vi "OE1022_Configure Ref Phase.vi"(7 "OE1022_Configure Ref Phase":T1={"Reference Source"=0, "Sweep Mode"=0, "Start Frequency(Hz)"=1000.0, "Stop Frequency(Hz)"=90000.0, "Linear Step Frequency(Hz)"=1000.0, "Log Step Percent(%)"=10.0, "Step Time(ms)"=1000, "Sweep Run Mode"=0, "Internal Frequency(Hz)"=1000.0, "Phase  (degree)"=0.0, "External Ref Trigger"=0} {"External Ref Trigger" items=["TTL Rising Edge", "TTL Falling Edge", "Sine Zero Crossing"]; "Phase  (degree)" min=-180.0 max=180.0 format="%.2f"; "Internal Frequency(Hz)" min=0.001 max=102000.0 format="%#.3f"; "Sweep Run Mode" items=["Stop", "Singal", "Loop"]; "Step Time(ms)" min=1 max=100000; "Log Step Percent(%)" min=0.0 max=100.0 format="%#.2g"; "Linear Step Frequency(Hz)" min=0.001 max=102000.0; "Stop Frequency(Hz)" min=0.001 max=102000.0 format="%#.3f"; "Start Frequency(Hz)" min=0.001 max=102000.0 format="%#.3f"; "Sweep Mode" items=["Linear", "Log"]; "Reference Source" items=["External", "Internal", "Internal Sweep"]}, 8 "Error in (no error)":errorcluster caption="error out（no error）", 9 "Remote Mode":u16(ring) items=["USB"=0, "GPIB"=2], 11 "VISA resource name":refnum<visa-resource-name>) -> (0 "Error out":errorcluster caption="error out", 1 "Output String":string, 3 "VISA resource  out":refnum<visa-resource-name>)   [LabVIEW 2011]
panel:
  out "字符串":string
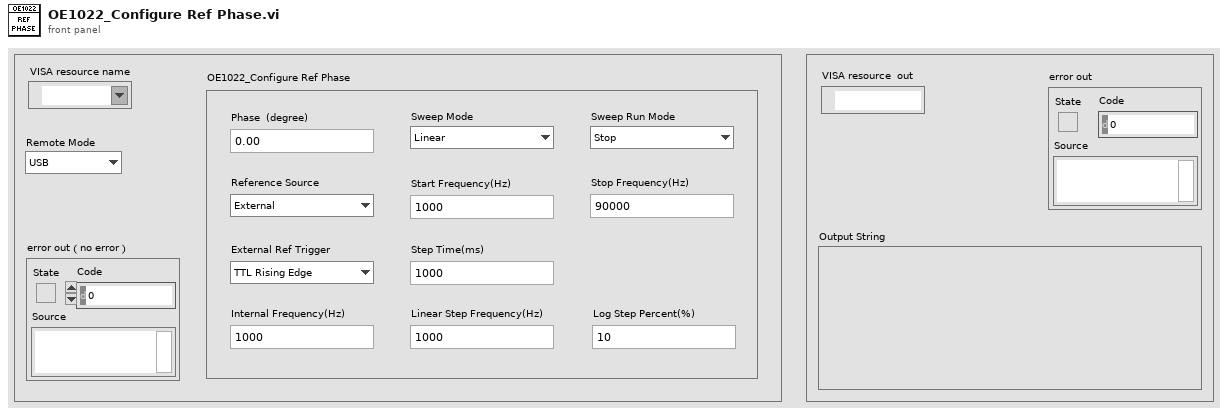
[diagram p1: front panel]
types:
  T1 = cluster{"Reference Source":u16, "Sweep Mode":u16, "Start Frequency(Hz)":dbl, "Stop Frequency(Hz)":dbl, "Linear Step Frequency(Hz)":dbl, "Log Step Percent(%)":dbl, "Step Time(ms)":i32, "Sweep Run Mode":u16, "Internal Frequency(Hz)":dbl, "Phase  (degree)":dbl, "External Ref Trigger":u16}
  T2 = enum16{"ISRC", "IGND", "ICPL", "ILIN", "PHAS", "FMOD", "RSLP", "FREQ", "SWPT", "SLLM", "SULM", "SSLL", "SSLG", "STLM", "SWRM", "IRNG", "SENS", "RMOD", "OFLT", "OFSL", "SYNC", "DMOD", "HARM", "DARB", "SWVT", "SLVL", "SVLL", "SVUL", "SVSL", "SVSG", "SVTM", "SVRM", "RALL", "SNAP", "OUTP", "OAUX", "COUT", "CAUX", "COFP", "CEXP", "FPOP", "OEXP", "*IDN", "*RST", "OVLD", "INOV", "GNOV", "*PLL", "SSET", "RSET", "AGAN", "APHS", "ARSV", "ASCL", "EQCD", "EQCS", "SPED", "SRAT", "SLEN", "SSLE", "STRG", "SPRM", "STRD", "PAUS", "REST", "SPTS", "TRCA", "TEMP", "RSTU", "IHNZ", "DEQU", "SADD", "ARNG", "CSPE", "ISRCD", "IGNDD", "ICPLD", "ILIND", "PHASD", "FMODD", "RSLPD", "FREQD", "SWPTD", "SLLMD", "SULMD", "SSLLD", "SSLGD", "STLMD", "SWRMD", "SENSD", "RMODD", "OFLTD", "OFSLD", "SYNCD", "HARMD", "EQCDD", "EQCSD", "SNAPD", "OUTPD", "SWVTD", "SLVLD", "SVLLD", "SVULD", "SVSLD", "SVSGD", "SVTMD", "SVRMD", "SVDCD", "ARSVD", "AGAND", "APHSD", "ASCLD", "FPOPD", "CAUXD", "OEXPD", "SPEDD", "SRATD", "SLEND", "SSLED", "STRGD", "SPRMD", "STRDD", "PAUSD", "RESTD", "SPTSD", "TRCAD", "*IDND", "*RSTD", "INOVD", "GNOVD", "*PLLD", "SSETD", "RSETD", "RALLD"}
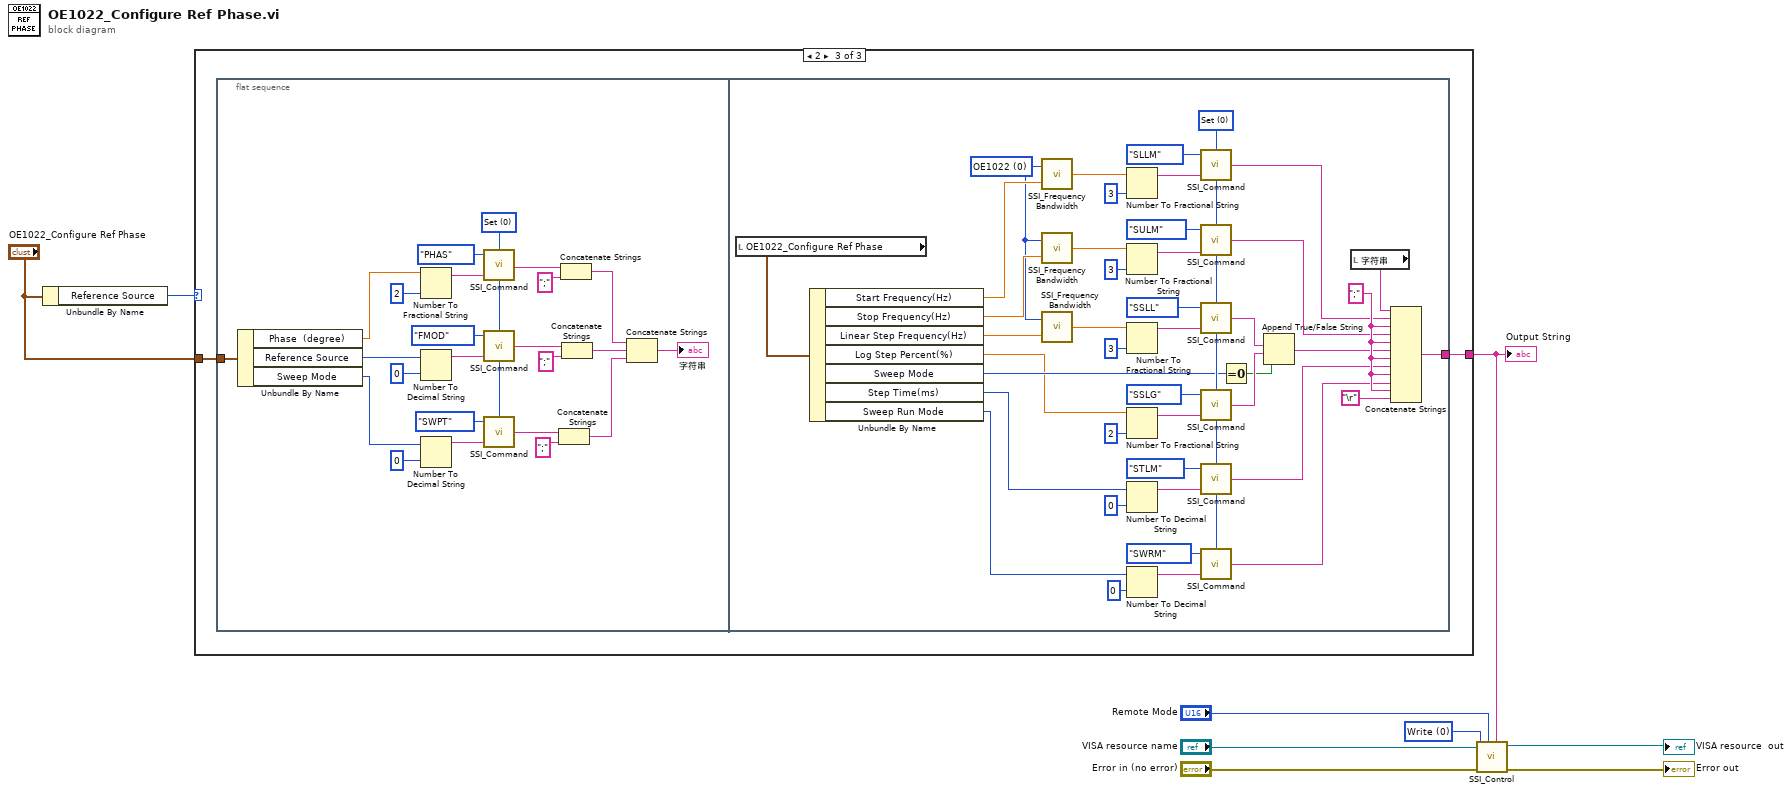
[diagram p0: block diagram]
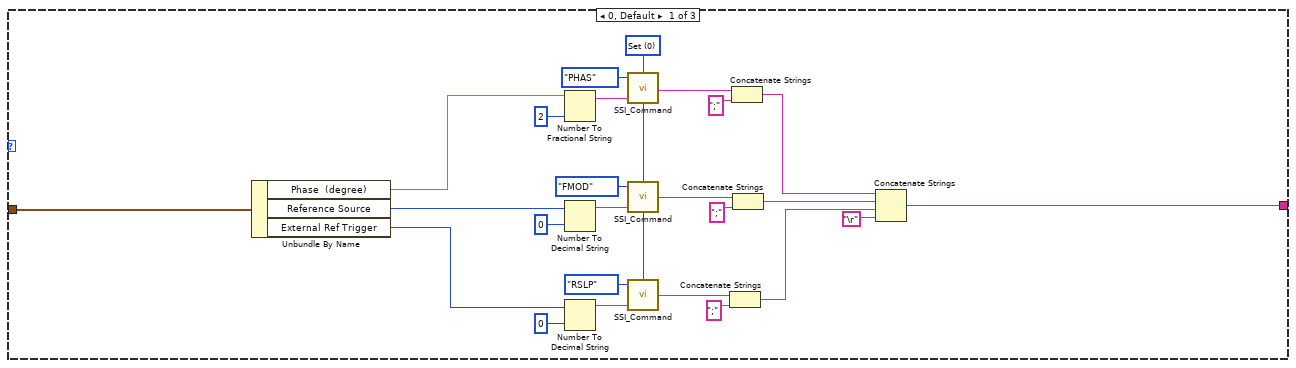
[diagram p2: hidden frame]
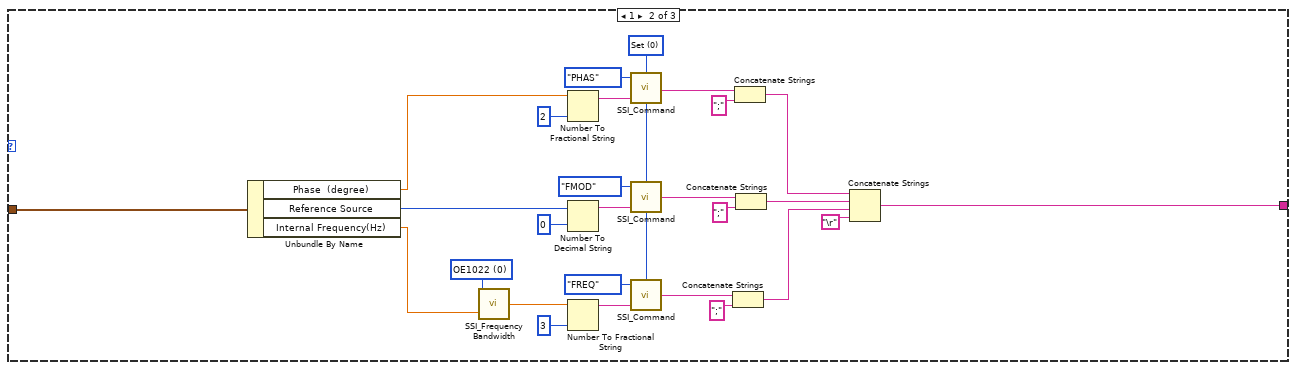
[diagram p3: hidden frame]
diagram:
  w9 = u16 0 items=["Write", "Read"] ("Control")
  n1 = Unbundle By Name("OE1022_Configure Ref Phase") -> ("Reference Source"=w3:u16)
  n2 = case shown="2" w3 {
    tunnel: "OE1022_Configure Ref Phase" -> [w21 w44 w63]
    tunnel: [w15 w43 w62] -> w1
    frame 0, Default {
      w20 = u16 0 items=["Set", "Query"] ("Opera")
      n3 = Unbundle By Name(w21) -> ("Phase  (degree)"=w10:dbl, "Reference Source"=w19:u16, "External Ref Trigger"=w22:u16)
      n4 = Number To Fractional String(number=w10, precision (6)=i16 2 ("精度(6)")) -> (F-format string=w33:string)  [unwired: 2 in]
      n5 = Number To Decimal String(number=w19, width (-)=i16 0 ("精度(6)")) -> (decimal integer string=w31:string)
      n6 = Number To Decimal String(number=w22, width (-)=i16 0 ("精度(6)")) -> (decimal integer string=w29:string)
      n7 = call "SSI_Command.vi"("Opera"=w20, "Paramter"=w33, "Command Type"=T2."PHAS") -> ("Output string"=w23:string)  [unwired: 1 in]
      n8 = call "SSI_Command.vi"("Opera"=w20, "Paramter"=w31, "Command Type"=T2."FMOD") -> ("Output string"=w25:string)  [unwired: 1 in]
      n9 = call "SSI_Command.vi"("Opera"=w20, "Paramter"=w29, "Command Type"=T2."RSLP") -> ("Output string"=w28:string)  [unwired: 1 in]
      n10 = Concatenate Strings(w28, ";" ("替换字符串(\"\")")) -> (w16:string)
      n11 = Concatenate Strings(w23, ";" ("替换字符串(\"\")")) -> (w18:string)
      n12 = Concatenate Strings(w25, ";" ("替换字符串(\"\")")) -> (w17:string)
      n13 = Concatenate Strings(w18, w17, w16, "\r") -> (w15:string)
    }
    frame 1 {
      w36 = u16 0 items=["OE1022", "OE1022D", "OE1201", "OE1311", "OE1351", "OE1301", "OE2031-10M", "OE2041-30M", "OE2041-60M"] ("Instrument Mode")
      w49 = u16 0 items=["Set", "Query"] ("Opera")
      n14 = Unbundle By Name(w44) -> ("Phase  (degree)"=w39:dbl, "Reference Source"=w48:u16, "Internal Frequency(Hz)"=w35:dbl)
      n15 = call "SSI_Frequency Bandwidth.vi"("Frequency"=w35, "Instrument Mode"=w36) -> ("Output"=w37:dbl)  [unwired: 1 in]
      n16 = Number To Fractional String(number=w39, precision (6)=i16 2 ("精度(6)")) -> (F-format string=w60:string)  [unwired: 2 in]
      n17 = Number To Decimal String(number=w48, width (-)=i16 0 ("精度(6)")) -> (decimal integer string=w58:string)
      n18 = Number To Fractional String(number=w37, precision (6)=i16 3 ("精度(6)")) -> (F-format string=w56:string)  [unwired: 2 in]
      n19 = call "SSI_Command.vi"("Opera"=w49, "Paramter"=w60, "Command Type"=T2."PHAS") -> ("Output string"=w50:string)  [unwired: 1 in]
      n20 = call "SSI_Command.vi"("Opera"=w49, "Paramter"=w58, "Command Type"=T2."FMOD") -> ("Output string"=w52:string)  [unwired: 1 in]
      n21 = call "SSI_Command.vi"("Opera"=w49, "Paramter"=w56, "Command Type"=T2."FREQ") -> ("Output string"=w55:string)  [unwired: 1 in]
      n22 = Concatenate Strings(w55, ";" ("替换字符串(\"\")")) -> (w45:string)
      n23 = Concatenate Strings(w50, ";" ("替换字符串(\"\")")) -> (w47:string)
      n24 = Concatenate Strings(w52, ";" ("替换字符串(\"\")")) -> (w46:string)
      n25 = Concatenate Strings(w47, w46, w45, "\r") -> (w43:string)
    }
    frame 2 {
      n26 = flat-sequence {
        tunnel: w63 -> [w69]
        tunnel: [w100] -> w62
        frame #0 {
          w74 = u16 0 items=["Set", "Query"] ("Opera")
          n27 = Unbundle By Name(w69) -> ("Phase  (degree)"=w67:dbl, "Reference Source"=w73:u16, "Sweep Mode"=w75:u16)
          n28 = Number To Fractional String(number=w67, precision (6)=i16 2 ("精度(6)")) -> (F-format string=w86:string)  [unwired: 2 in]
          n29 = Number To Decimal String(number=w73, width (-)=i16 0 ("精度(6)")) -> (decimal integer string=w84:string)
          n30 = Number To Decimal String(number=w75, width (-)=i16 0 ("精度(6)")) -> (decimal integer string=w82:string)
          n31 = call "SSI_Command.vi"("Opera"=w74, "Paramter"=w86, "Command Type"=T2."PHAS") -> ("Output string"=w76:string)  [unwired: 1 in]
          n32 = call "SSI_Command.vi"("Opera"=w74, "Paramter"=w84, "Command Type"=T2."FMOD") -> ("Output string"=w78:string)  [unwired: 1 in]
          n33 = call "SSI_Command.vi"("Opera"=w74, "Paramter"=w82, "Command Type"=T2."SWPT") -> ("Output string"=w81:string)  [unwired: 1 in]
          n34 = Concatenate Strings(w81, ";" ("替换字符串(\"\")")) -> (w70:string)
          n35 = Concatenate Strings(w76, ";" ("替换字符串(\"\")")) -> (w72:string)
          n36 = Concatenate Strings(w78, ";" ("替换字符串(\"\")")) -> (w71:string)
          n37 = Concatenate Strings(w72, w71, w70) -> (→"字符串":string)
        }
        frame #1 {
          w89 = u16 0 items=["OE1022", "OE1022D", "OE1201", "OE1311", "OE1351", "OE1301", "OE2031-10M", "OE2041-30M", "OE2041-60M"] ("Instrument Mode")
          w130 = ";"
          w120 = u16 0 items=["Set", "Query"] ("Opera")
          n38 = local read "OE1022_Configure Ref Phase"() -> (w90:T1)
          n39 = Unbundle By Name(w90) -> ("Start Frequency(Hz)"=w104:dbl, "Stop Frequency(Hz)"=w103:dbl, "Linear Step Frequency(Hz)"=w102:dbl, "Log Step Percent(%)"=w88:dbl, "Sweep Mode"=w99:u16, "Step Time(ms)"=w98:i32, "Sweep Run Mode"=w97:u16)
          n40 = call "SSI_Frequency Bandwidth.vi"("Frequency"=w104, "Instrument Mode"=w89) -> ("Output"=w107:dbl)  [unwired: 1 in]
          n41 = call "SSI_Frequency Bandwidth.vi"("Frequency"=w103, "Instrument Mode"=w89) -> ("Output"=w106:dbl)  [unwired: 1 in]
          n42 = call "SSI_Frequency Bandwidth.vi"("Frequency"=w102, "Instrument Mode"=w89) -> ("Output"=w105:dbl)  [unwired: 1 in]
          n43 = Number To Fractional String(number=w107, precision (6)=i16 3 ("精度(6)")) -> (F-format string=w116:string)  [unwired: 2 in]
          n44 = Number To Fractional String(number=w106, precision (6)=i16 3 ("精度(6)")) -> (F-format string=w114:string)  [unwired: 2 in]
          n45 = Number To Fractional String(number=w105, precision (6)=i16 3 ("精度(6)")) -> (F-format string=w112:string)  [unwired: 2 in]
          n46 = Number To Fractional String(number=w88, precision (6)=i16 2 ("精度(6)")) -> (F-format string=w110:string)  [unwired: 2 in]
          n47 = Number To Decimal String(number=w98, width (-)=i16 0 ("精度(6)")) -> (decimal integer string=w108:string)
          n48 = Number To Decimal String(number=w97, width (-)=i16 0 ("精度(6)")) -> (decimal integer string=w118:string)
          n49 = call "SSI_Command.vi"("Opera"=w120, "Paramter"=w116, "Command Type"=T2."SLLM") -> ("Output string"=w124:string)  [unwired: 1 in]
          n50 = call "SSI_Command.vi"("Opera"=w120, "Paramter"=w114, "Command Type"=T2."SULM") -> ("Output string"=w125:string)  [unwired: 1 in]
          n51 = call "SSI_Command.vi"("Opera"=w120, "Paramter"=w112, "Command Type"=T2."SSLL") -> ("Output string"=w122:string)  [unwired: 1 in]
          n52 = call "SSI_Command.vi"("Opera"=w120, "Paramter"=w110, "Command Type"=T2."SSLG") -> ("Output string"=w123:string)  [unwired: 1 in]
          n53 = call "SSI_Command.vi"("Opera"=w120, "Paramter"=w108, "Command Type"=T2."STLM") -> ("Output string"=w127:string)  [unwired: 1 in]
          n54 = call "SSI_Command.vi"("Opera"=w120, "Paramter"=w118, "Command Type"=T2."SWRM") -> ("Output string"=w128:string)  [unwired: 1 in]
          n55 = Equal To 0?(x=w99) -> (x = 0?=w121:bool)
          n56 = Append True/False String(1:w121, 2:w123, 3:w122) -> (0:w126:string)  [unwired: 1 in]
          n57 = local read "字符串"() -> (w101:string)
          n58 = Concatenate Strings(w101, w124, w130, w125, w130, w126, w130, w127, w130, w128, w130, "\r") -> (w100:string)
        }
      }
    }
  }
  "Output String" <- w1
  n59 = call "SSI_Control.vi"("Write Buffer"=w1, "Remote Mode"="Remote Mode", "Error in (no error)"="Error in (no error)", "Control"=w9, "VISA resource name"="VISA resource name") -> ("Error out"=→"Error out":errorcluster, "VISA resource  out"=→"VISA resource  out":refnum<visa-resource-name>)  [unwired: 3 in, 2 out]
